vi "Pfeiffer Vacuum Turbo Miscellaneous.vi"(8 "error in (no error)":errorcluster, 9 "PV Miscellaneous - Cluster":T1={"Parameter"=enum." Preselection brake", "Parameter\nread only<->describe"=FALSE, "off<->on   "=TRUE, "Unit adress"=1, "Contens of service\nline; # of the 2nd\n parameter"=0} {"Unit adress" min=1 max=255 step=1}, 10 "Adress of unit":u16=1 min=1 max=999 step=1, 11 "COM Port Name in":refnum<visa-resource-name>="COM1") -> (0 "error out":errorcluster, 3 "response (data)":string)   [LabVIEW 2021]
doc: "This VI is an example of how to use the Pfeiffer Vacuum subVIs programmatically. This VI first initializes the instrument, takes measurements, then closes the instrument."
uses:
  <instrlib>/Pfeiffer Vacuum/Public/Turbopumps/PV Miscellaneous - Cluster.ctl
  <instrlib>/Pfeiffer Vacuum/Pfeiffer Vacuum.lvlib
panel:
  # "Preselection brake             :  \n Remote operations mode  : \n Configuration output K4    : \n Parameter set                      :\n Seal gas enable                   :\n Keyboard interlock            :"
  # "<--------------\n  off\n  stand. operations \n  heat/TMS\n  basic  \n  off\n  off"
  # "----------->          \non \nremote priority \nPWM-signal \n extended \non \non"
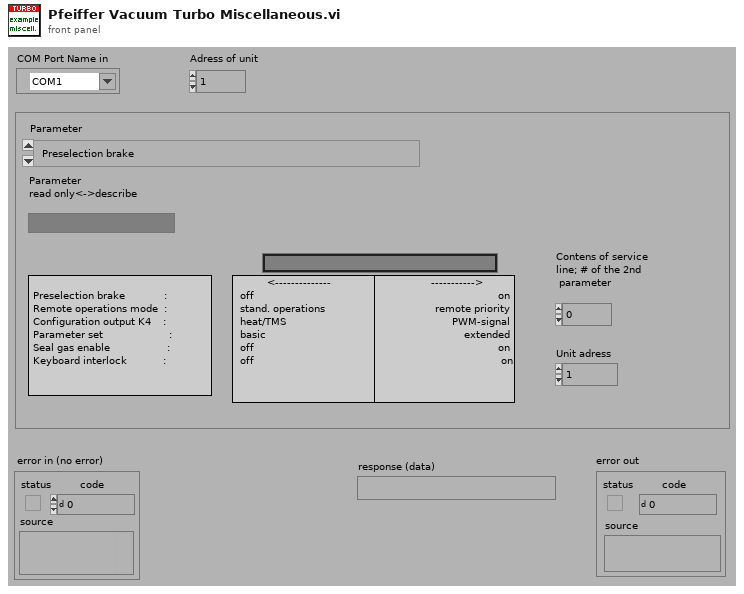
[diagram p1: front panel]
types:
  T1 = typedef "Pfeiffer Vacuum.lvlib/PV Miscellaneous - Cluster.ctl" = cluster{"Parameter":enum16{" Preselection brake", " Remote operations mode", " Actual error code (read only)", " Software version electronic drive unit  (read only)", " Software version display and control unit  (read only)", " Parameter set", " Contens of service line (TCM 1601 only)", " Unit adress", " Unit type electronic drive unit", " Error acknowledgement (write only)", " Keyboard interlock (008)", " Seal gas enable (050)"}, "Parameter\nread only<->describe":bool, "off<->on   ":bool, "Unit adress":i16, "Contens of service\nline; # of the 2nd\n parameter":i16}
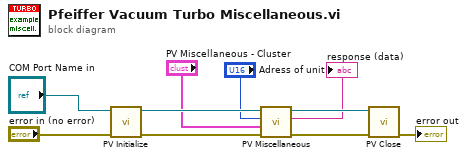
[diagram p0: block diagram]
diagram:
  n1 = call <instrlib>:"PV Initialize.vi"("error in (no error)"="error in (no error)", "VISA session in"="COM Port Name in") -> ("error out"=w10:errorcluster, "VISA session out"=w8:refnum<visa-resource-name>)  [unwired: 8 in]
  n2 = call <instrlib>:"PV Miscellaneous.vi"("error in (no error)"=w10, "PV Miscellaneous - Cluster"="PV Miscellaneous - Cluster", "Adress of unit"="Adress of unit", "VISA session"=w8) -> ("error out"=w9:errorcluster, "response (data)"=→"response (data)":string, "dup VISA session"=w7:refnum<visa-resource-name>)  [unwired: 5 in]
  n3 = call <instrlib>:"PV Close.vi"("VISA session"=w7, "error in (no error)"=w9) -> ("error out"=→"error out":errorcluster)  [unwired: 13 in]
